vi "Write Data to the PI System via OMF (v1.0).vi"() -> ()   [LabVIEW 2014]
uses:
  <vilib>/Platform/TimedLoop/XDataNode/timing_clust.ctl
  <vilib>/Platform/TimedLoop/XDataNode/nitl_modes.ctl
  <vilib>/Platform/TimedLoop/XDataNode/wakeup.ctl
  <vilib>/platform/TimedLoop/XDataNode/XDataNode.xnode
  <vilib>/Platform/TimedLoop/XDataNode/XDNodeRunTimeDep.lvlib
panel:
  in  "Stop looping":bool
  in  "OMF Static Type Instance Name":string="LabVIEW AF Element 6"
  out "Response body for initial OMF messages":string
  out "Reponse headers for initial OMF messages":string
  out "Number of continuous OMF data messages sent":i32
  out "Reponse body for continuous OMF data messages":string
  out "Response headers for continuous OMF data messages":string
  out "error out":errorcluster
  in  "Allow untrusted certificates?":bool=TRUE
  in  "OMF Dynamic Type Property Names and Formats":T1(array[cluster])=[{"Dynamic Property Name"="X acceleration", "Dynamic Property Format"=enum."number"}, {"Dynamic Property Name"="Y acceleration", "Dynamic Property Format"=enum."number"}, {"Dynamic Property Name"="Z acceleration", "Dynamic Property Format"=enum."number"}, {"Dynamic Property Name"="Heartbeat Tag (String)", "Dynamic Property Format"=enum."string"}]
  in  "OMF Static Type Property Names, Formats, and Values":T2(array[cluster])=[{"Static Property Name"="Data ingress method", "Static Property Format"=enum."string", "Static Property Value"="\"OMF\""}, {"Static Property Name"="Version", "Static Property Format"=enum."number", "Static Property Value"="1"}]
  in  "Seconds in between continuous data messages":i32=1
  in  "OMF Static Type ID":string="LabVIEW Static Type 6"
  in  "OMF Dynamic Type ID":string="LabVIEW Dynamic Type 6"
  in  "OMF Container ID":string="LabVIEW Data Container 6"
  in  "OMF Producer Token":string="uid=41570fd7-1a7c-46fc-a6c0-c03aa973fdd2&sig=az5RilkdL6Nq2qgkj64lNRau6M8X59LDLitGKMfWFUM="
  in  "OMF Ingress URL":string="https://dloserver2016r2:8118/ingress/messages"
  # "Configuration"
  # "Response Messages"
  # "Note: if the response header is \"HTTP/1.1 204 No Content\" and the response body is empty, that indicates that a message was received successfully!"
  # "Note: the OMF Ingress URL and OMF Producer Token can be obtained from within the PI Data Collection Manager"
  # "(Stop sending continuous messages)"
  # "Note: If you are testing against a stock installation, one that still uses an untructed, self-signed certificate (which is the default), set this to \"ON\""
  # "Note: the Static Type Instance Name (below) will be the name of the PI AF Element that is created on the target PI System"
  # "Error Messages"
  # "Note: when specifying the value for a static property (above), if the property format is \"string\" add double quotes around the string value; if the property format \"number\", do not add double quotes around the numeric value."
  # "Note: remember the order in which you specify these dynamic properties! Later within your VI, you will wire in a string array of live data values for these dynamic properties, and the order of values in that array must match the order of properties that you specify above (i.e., if you listed that the first property is \"X acceleration\", you need to make sure that the first value in your string array is the x acceleration value)."
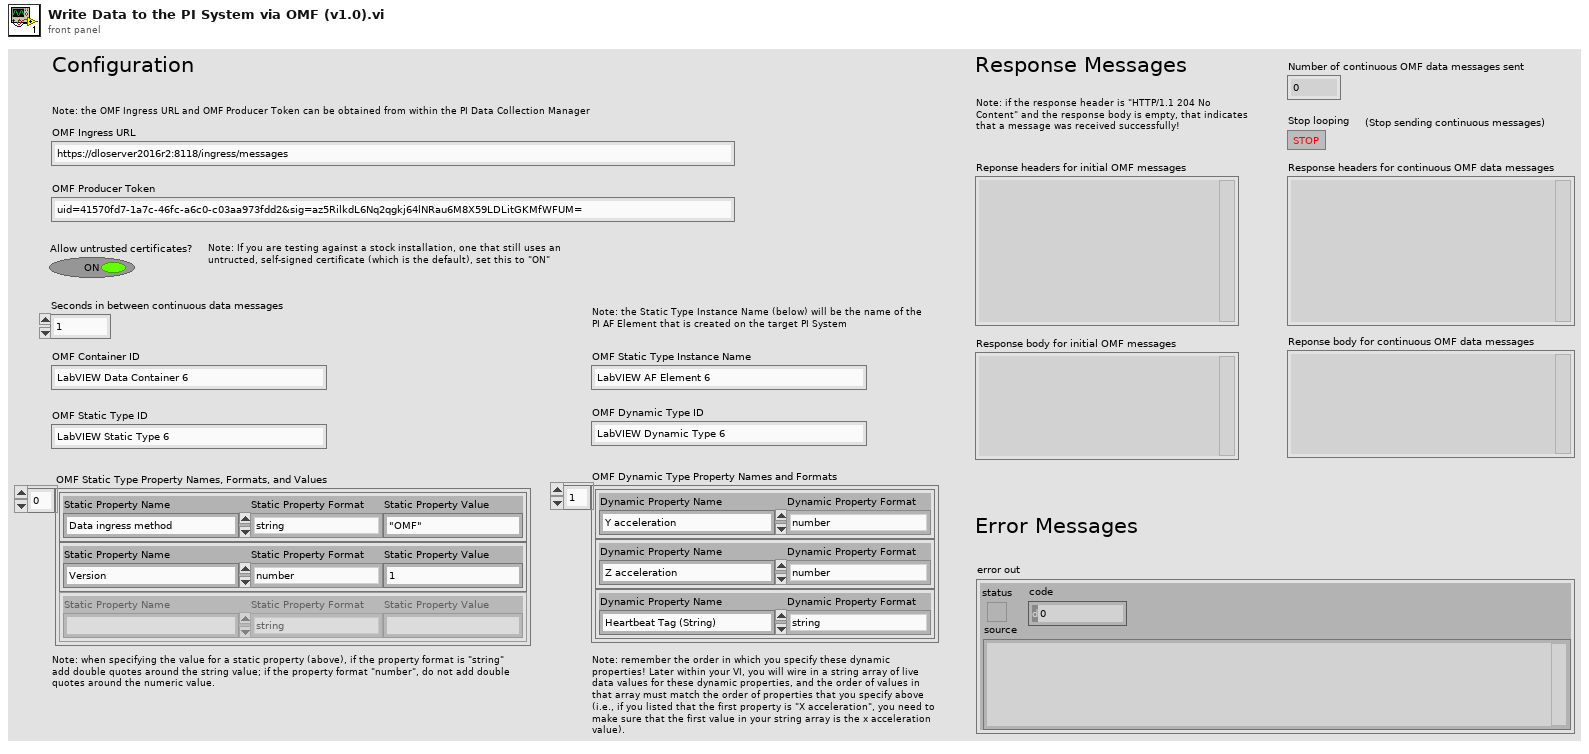
[diagram p1: front panel]
types:
  T1 = cluster{"Dynamic Property Name":string, "Dynamic Property Format":enum16{"string", "number"}}[]
  T2 = cluster{"Static Property Name":string, "Static Property Format":enum16{"string", "number"}, "Static Property Value":string}[]
  T3 = typedef "LabVIEWHTTPClient.lvlib/ClientHandle.ctl" = refnum<k1>
  T4 = typedef "XDNodeRunTimeDep.lvlib/timing_clust.ctl" = cluster{"Expected End [f-1]":u64, "Actual End [f-1]":u64, "Finished Late? [f-1]":bool, "Expected End [i-1]":u64, "Actual End [i-1]":u64, "Finished Late? [i-1]":bool, "Expected Start [i]":u64, "Actual Start [i]":u64, "Expected Start [f]":u64, "Actual Start [f]":u64, "Source Name":string, "Structure Name":string, "Period":i64, "Deadline":i64, "Offset":i64, "Start":i64, "Priority":i32, "Timeout":i32, "Mode":T5, "Wakeup Reason":T6, "Error":errorcluster, "Source Type":string, "Secondary Source Type":string, "Global End Time":u64, "Global Start Time":u64, "Frame Duration":u64, "Iteration Duration":u64, "Assigned CPU":i32, "I/O Scan Engine Mode":u32}
  T5 = typedef "XDNodeRunTimeDep.lvlib/nitl_modes.ctl" = enum32{"No Change", "Process missed periods, maintain original phase", "Discard missed periods, maintain original phase", "Process missed periods, ignore original phase", "Discard missed periods, ignore original phase"}
  T6 = typedef "XDNodeRunTimeDep.lvlib/wakeup.ctl" = enum32{"Normal", "Aborted", "Asynchronous wakeup", "Timing source error", "Timed loop error", "Timeout"}
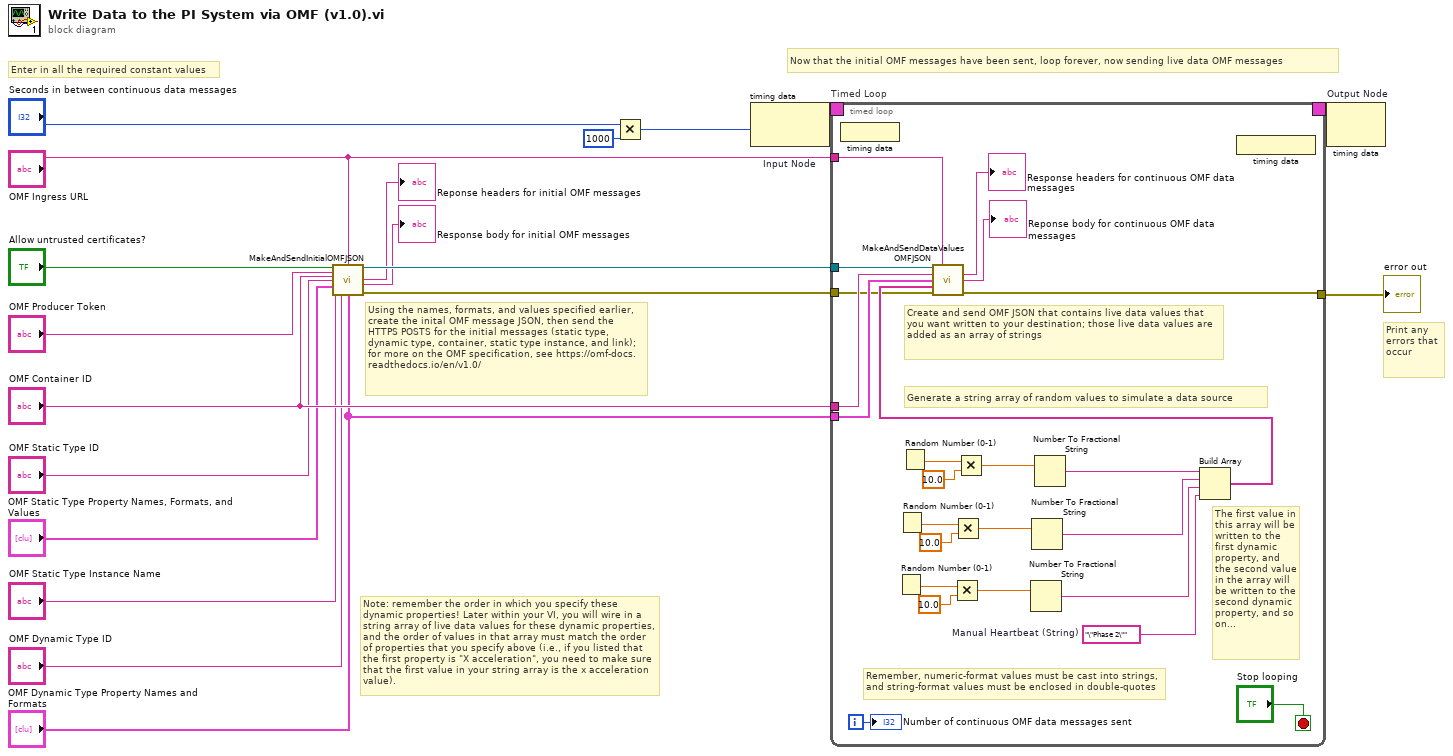
[diagram p0: block diagram]
diagram:
  # "Note: remember the order in which you specify these dynamic properties! Later within your VI, you will wire in a string array of live data values for these dynamic properties, and the order of values in that array must match the order of properties that you specify above (i.e., if you listed that the first property is \"X acceleration\", you need to make sure that the first value in your string array is the x acceleration value)."
  # "Now that the initial OMF messages have been sent, loop forever, now sending live data OMF messages"
  # "Using the names, formats, and values specified earlier, create the inital OMF message JSON, then send the HTTPS POSTS for the initial messages (static type, dynamic type, container, static type instance, and link); for more on the OMF specification, see https://omf-docs.readthedocs.io/en/v1.0/"
  # "Print any errors that occur"
  # "Enter in all the required constant values"
  n1 = call "MakeAndSendInitialOMFJSON.vi"("Allow untrusted certificates?"="Allow untrusted certificates?", "OMF Producer Token"="OMF Producer Token", "OMF Ingress URL"="OMF Ingress URL", "OMF Container ID"="OMF Container ID", "OMF Static Type ID"="OMF Static Type ID", "OMF Static Type Property Names, Formats, and Values"="OMF Static Type Property Names, Formats, and Values", "OMF Static Type Instance Name"="OMF Static Type Instance Name", "OMF Dynamic Type ID"="OMF Dynamic Type ID", "OMF Dynamic Type Property Names and Formats"="OMF Dynamic Type Property Names and Formats") -> ("client handle out"=w10:T3, "Reponse headers for initial OMF messages"=→"Reponse headers for initial OMF messages":string, "Response body for initial OMF messages"=→"Response body for initial OMF messages":string, "error out"=w9:errorcluster)  [unwired: 3 in]
  n2 = Multiply(x="Seconds in between continuous data messages", y=1000) -> (x*y=w14:i32)
  n3 = node-c288 "Input Node"(w14) -> (w18:T4)
  n4 = timed-loop "Timed Loop" {
    timing: w18 -> [_]
    timing-out: [_] -> w17
    tunnel: w10 -> [w26]
    tunnel: "OMF Ingress URL" -> [w25]
    tunnel: w9 -> [w27]
    tunnel: [w22] -> w19
    tunnel: "OMF Container ID" -> [w29]
    tunnel: "OMF Dynamic Type Property Names and Formats" -> [w30]
    i -> [w43]
    stop <- "Stop looping" stop-if-true
    w20 = "\"Phase 2\""  # Manual Heartbeat (String)
    # "Remember, numeric-format values must be cast into strings, and string-format values must be enclosed in double-quotes"
    # "The first value in this array will be written to the first dynamic property, and the second value in the array will be written to the second dynamic property, and so on..."
    # "Generate a string array of random values to simulate a data source"
    # "Create and send OMF JSON that contains live data values that you want written to your destination; those live data values are added as an array of strings"
    n5 = node-c288 ("Output Node")() -> ()  [unwired: 1 in]
    n6 = Random Number (0-1)() -> (number: 0 to 1=w35:dbl)
    n7 = Random Number (0-1)() -> (number: 0 to 1=w38:dbl)
    n8 = Random Number (0-1)() -> (number: 0 to 1=w42:dbl)
    n9 = Multiply(x=w35, y=10.0) -> (x*y=w33:dbl)
    n10 = Multiply(x=w38, y=10.0) -> (x*y=w36:dbl)
    n11 = Multiply(x=w42, y=10.0) -> (x*y=w40:dbl)
    n12 = Number To Fractional String(number=w33) -> (F-format string=w31:string)  [unwired: 3 in]
    n13 = Number To Fractional String(number=w36) -> (F-format string=w32:string)  [unwired: 3 in]
    n14 = Number To Fractional String(number=w40) -> (F-format string=w39:string)  [unwired: 3 in]
    n15 = Build Array "Build Array"(w39, w32, w31, w20) -> (w28:string[])
    n16 = call "MakeAndSendDataValuesOMFJSON.vi"("client handle"=w26, "OMF Ingress URL"=w25, "OMF Container ID"=w29, "OMF Dynamic Type Property Names and Formats"=w30, "Array of Values"=w28, "error in (no error)"=w27) -> ("Response headers for continuous OMF data messages"=→"Response headers for continuous OMF data messages":string, "Reponse body for continuous OMF data messages"=→"Reponse body for continuous OMF data messages":string, "error out"=w22:errorcluster)  [unwired: 7 in]
    n17 = node-c288() -> ()  [unwired: 1 out]
    "Number of continuous OMF data messages sent" <- w43
  }
  "error out" <- w19
  n18 = node-c288 "Output Node"(w17) -> ()  [unwired: 1 out]
